vi "Pressure_Jog_Z.vi"() -> (3 "current Z":sgl)   [LabVIEW 2013]
uses:
  <vilib>/Analysis/baseanly.llb/Mean (DBL).vi
  <vilib>/LabVIEW Interface for Arduino/LabVIEW Interface for Arduino.lvlib
  <vilib>/Analysis/NI_AALBase.lvlib
panel:
  out "Current Z Position":sgl
  in  "MG17Motor":refnum<k7>(container)
  in  "Serial":i32=90848557
  out "Force Threshhold Reached":bool
  out "Force Average":dbl format="%0.2f"
  out "Force vs Time":dbl(graph)
  out "Voltage Average":dbl format="%0.2f"
  in  "Array":dbl[](array[numeric])
  in  "Analog Input Pin":u8
  in  "Stop":bool
  out "Volatege vs Time":dbl(graph)
  out "output array":dbl[](array[numeric])
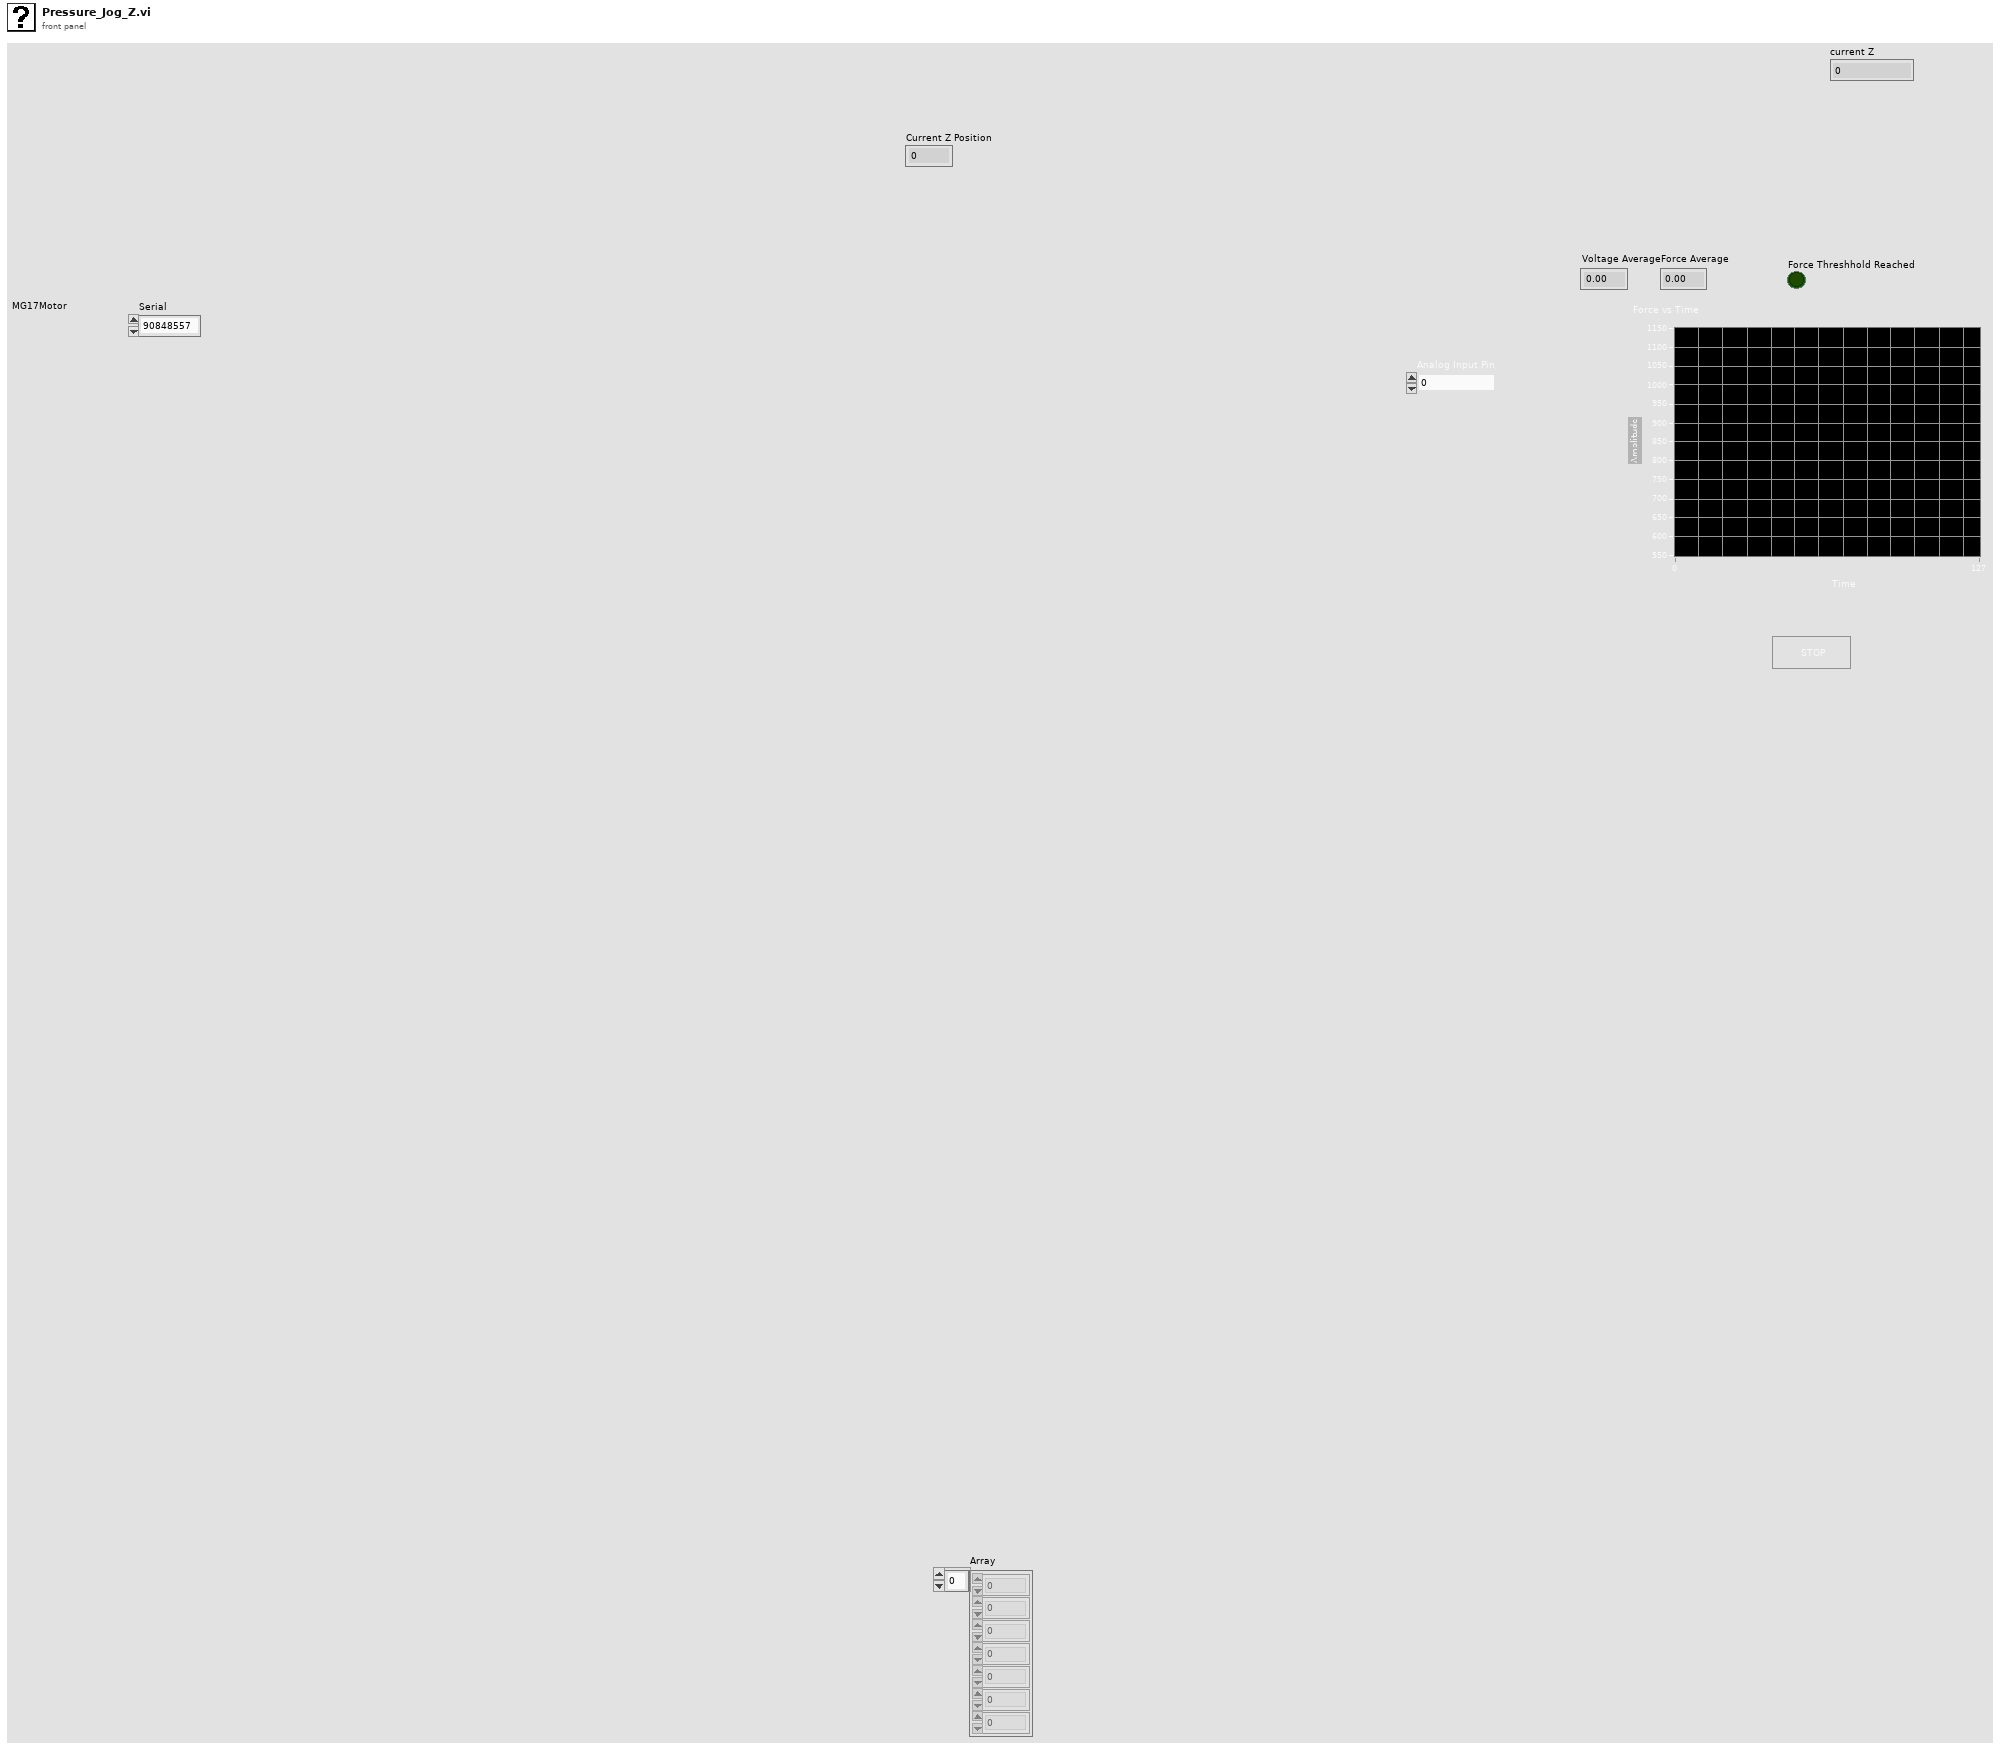
[diagram p1: front panel]
types:
  T1 = typedef "LabVIEW Interface for Arduino.lvlib/Arduino Resource.ctl" = cluster{"VISA resource":refnum<visa-resource-name>, "Board Type":T2, "Connection Type":enum8{"USB / Serial"}, "Bytes Per Packet (15)":u8}
  T2 = typedef "LabVIEW Interface for Arduino.lvlib/Board Type.ctl" = enum16{"Uno", "Dimuelanove w/Atmega 328", "Mega 2560"}
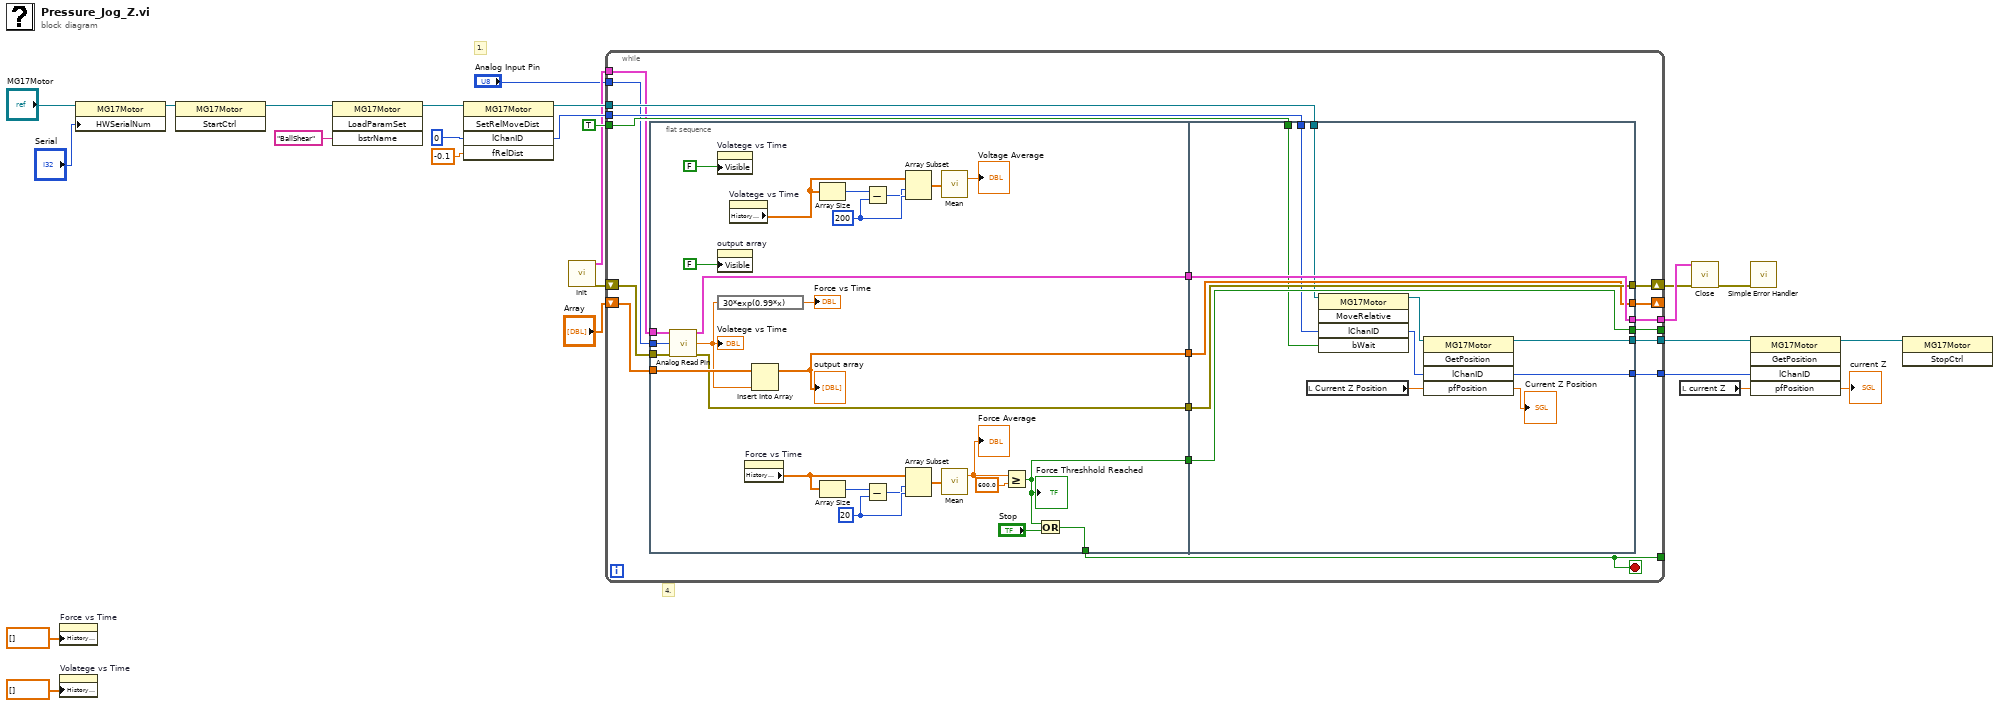
[diagram p0: block diagram]
diagram:
  # "4."
  # "1."
  n1 = property on="Force vs Time" class="WFChart (strict)"("History Data"=dbl[] []) -> ()  [unwired: 2 in, 2 out]
  n2 = property on="Volatege vs Time" class="WFChart (strict)"("History Data"=dbl[] []) -> ()  [unwired: 2 in, 2 out]
  n3 = property class="MG17Motor"(reference="MG17Motor", "HWSerialNum"="Serial") -> (reference out=w19:refnum<k7>)  [unwired: 1 in, 1 out]
  n4 = invoke class="MG17Motor" method="StartCtrl"(reference=w19) -> (reference out=w18:refnum<k7>)  [unwired: 2 in, 2 out]
  n5 = invoke class="MG17Motor" method="LoadParamSet"(reference=w18, "bstrName"="BallShear") -> (reference out=w14:refnum<k7>)  [unwired: 2 in, 3 out]
  n6 = invoke class="MG17Motor" method="SetRelMoveDist"(reference=w14, "lChanID"=0, "fRelDist"=-0.1) -> (reference out=w11:refnum<k7>, "lChanID"=w10:i32)  [unwired: 2 in, 3 out]
  n7 = call <vilib>:"Init.vi"() -> ("Arduino Resource"=w8:T1, "error out"=w6:errorcluster)  [unwired: 18 in]
  n8 = while {
    tunnel: [w43] -> w25
    shift-right: [w42] -> w23
    shift-left: w6 -> [w41]
    shift-right: [w39] -> _
    shift-left: "Array" -> [w40]
    tunnel: [w38] -> _
    tunnel: [w37] -> _
    tunnel: w11 -> [w32]
    tunnel: w10 -> [w31]
    tunnel: [w30] -> w5
    tunnel: TRUE -> [w29]
    tunnel: w8 -> [w28]
    tunnel: "Analog Input Pin" -> [w27]
    tunnel: [w26] -> w1
    stop <- w37 stop-if-true
    n9 = flat-sequence {
      tunnel: w41 -> [w45]
      tunnel: w40 -> [w70]
      tunnel: [w50] -> w37
      tunnel: [w47] -> w36
      tunnel: [w46] -> w35
      tunnel: [w69] -> w34
      tunnel: [w51] -> w33
      tunnel: w28 -> [w49]
      tunnel: w27 -> [w48]
      tunnel: [w80] -> w38
      tunnel: [w81] -> w39
      tunnel: [w82] -> w42
      tunnel: [w83] -> w43
      tunnel: w36 -> [w83]
      tunnel: w35 -> [w82]
      tunnel: w34 -> [w81]
      tunnel: w33 -> [w80]
      tunnel: w32 -> [w76]
      tunnel: w31 -> [w75]
      tunnel: [w74] -> w30
      tunnel: w29 -> [w73]
      tunnel: [w71] -> w26
      frame #0 {
        w61 = 200 ("length")
        w58 = 20 ("length")
        n10 = call <vilib>:"Analog Read Pin.vi"("Arduino Resource"=w49, "Analog Input Pin (0)"=w48, "error in"=w45) -> ("Arduino Resource"=w47:T1, "Voltage"=w44:dbl, "error out"=w46:errorcluster)  [unwired: 10 in]
        "Volatege vs Time" <- w44
        n11 = property on="Volatege vs Time" class="WFChart (strict)"("Visible"=FALSE) -> ()  [unwired: 2 in, 2 out]
        n12 = property on="output array" class="Arr (strict)"("Visible"=FALSE) -> ()  [unwired: 2 in, 2 out]
        n13 = expression code="30*exp(0.99*x)"(w44) -> (→"Force vs Time":dbl)
        n14 = property on="Volatege vs Time" class="WFChart (strict)"() -> ("History Data"=w65:dbl[])  [unwired: 2 in, 2 out]
        n15 = property on="Force vs Time" class="WFChart (strict)"() -> ("History Data"=w67:dbl[])  [unwired: 2 in, 2 out]
        n16 = Insert Into Array(array=w70, new element=w44) -> (w69:dbl[])  [unwired: 1 in]
        "output array" <- w69
        n17 = Array Size(array=w65) -> (size(s)=w62:i32)
        n18 = Array Size(array=w67) -> (size(s)=w59:i32)
        n19 = Subtract(x=w62, y=w61) -> (x-y=w60:i32)
        n20 = Subtract(x=w59, y=w58) -> (x-y=w57:i32)
        n21 = Array Subset(array=w65, index=w60, length=w61) -> (w63:dbl[])
        n22 = Array Subset(array=w67, index=w57, length=w58) -> (w66:dbl[])
        n23 = call-poly <vilib>:"Mean.vi"("X"=w63) -> ("mean"=→"Voltage Average":dbl)  [unwired: 1 out]
        n24 = call-poly <vilib>:"Mean.vi"("X"=w66) -> ("mean"=w56:dbl)  [unwired: 1 out]
        "Force Average" <- w56
        n25 = Greater Or Equal?(x=w56, y=600.0) -> (x >= y?=w51:bool)
        "Force Threshhold Reached" <- w51
        n26 = Or(x=w51, y="Stop") -> (x .or. y?=w50:bool)
      }
      frame #1 {
        n27 = local read "Current Z Position"() -> (w72:sgl)
        n28 = invoke class="MG17Motor" method="MoveRelative"(reference=w76, "lChanID"=w75, "bWait"=w73) -> (reference out=w77:refnum<k7>, "lChanID"=w78:i32)  [unwired: 2 in, 3 out]
        n29 = invoke class="MG17Motor" method="GetPosition"(reference=w77, "lChanID"=w78, "pfPosition"=w72) -> (reference out=w74:refnum<k7>, "lChanID"=w71:i32, "pfPosition"=→"Current Z Position":sgl)  [unwired: 2 in, 2 out]
      }
    }
  }
  n30 = local read "current Z"() -> (w3:sgl)
  n31 = call <vilib>:"Close.vi"("Arduino Resource"=w25, "error in"=w23) -> ("error out"=w24:errorcluster)  [unwired: 13 in]
  n32 = call <vilib>:"Simple Error Handler.vi"("error in (no error)"=w24) -> ()  [unwired: 4 in, 5 out]
  n33 = invoke class="MG17Motor" method="GetPosition"(reference=w5, "lChanID"=w1, "pfPosition"=w3) -> (reference out=w4:refnum<k7>, "pfPosition"=→"current Z":sgl)  [unwired: 2 in, 3 out]
  n34 = invoke class="MG17Motor" method="StopCtrl"(reference=w4) -> ()  [unwired: 2 in, 3 out]
